vi "Write Sample Container.vi"(8 "error in (no error)":errorcluster, 10 "Sample Container":T1, 11 "Syringe in":refnum<class "Syringe Line.lvclass">) -> (0 "error out":errorcluster, 3 "Syringe out":refnum<class "Syringe Line.lvclass">)   [LabVIEW 2015, in "cRIO-Carbondioxide.lvlib" / "CO2-Actor.lvlib" / "Syringe Line.lvclass"]
uses:
  Syringe Line.lvclass
  Controls/Sample Container.ctl
  subs/Sample/Sample.lvclass
  Syringe Line.lvclass/Syringe Line.ctl
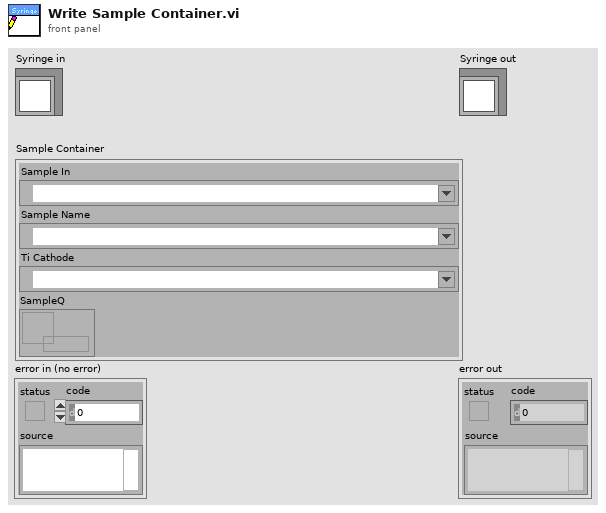
[diagram p1: front panel]
types:
  T1 = typedef "Sample Container.ctl" = cluster{"Sample In":refnum<k21>, "Sample Name":refnum<k21>, "Ti Cathode":refnum<k21>, "SampleQ":refnum<queue>}
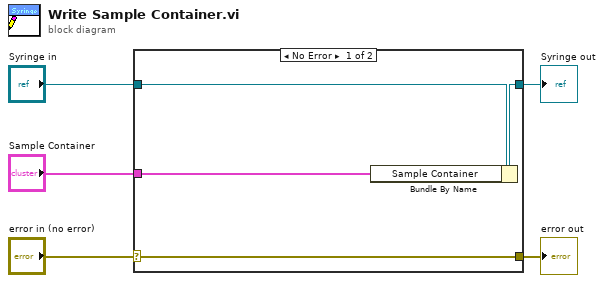
[diagram p0: block diagram]
diagram:
  n1 = case shown="No Error" "error in (no error)" {
    selector: "error in (no error)" -> [w9 w10]
    tunnel: [w9 w10] -> w4
    tunnel: [w7 w11] -> w2
    tunnel: "Syringe in" -> [w8 w11]
    tunnel: "Sample Container" -> [w6 _]
    frame No Error {
      n2 = Bundle By Name(cluster=w8, "Sample Container"=w6) -> (w7:refnum<class "Syringe Line.lvclass">)
    }
    frame Error {
    }
  }
  "error out" <- w4
  "Syringe out" <- w2
